vi "Read Section Cluster.vi"(6 "Section (Cluster Name)":string, 7 "error in (no error)":errorcluster, 8 "Cluster":variant, 9 "Offset":i32, 10 "JSON Object":string="{}") -> (0 "error out":errorcluster, 1 "Cluster set from section":variant, 2 "Section Found":bool)   [LabVIEW 2015, in "JSONtext.lvlib"]
doc: "Set the value of a Section Cluster from a Section of a JSON object. If the Section is not specified, then the data name of the Cluster will be used.\n\nA \"Section Cluster\" is defined in analogy to the OpenG Variant Config Library \"Section Cluster\" functions, using a JSON Object, with subObjects representing \"Sections\", instead of INI format."
uses:
  JSONtext.lvlib
  Find Object Item (single) by Path.vi
  String Subset.vi
  Find Item Locations by Path.vi
  JSON text to Variant.vi
  <vilib>/Utility/Data Type/NI_Data Type.lvlib
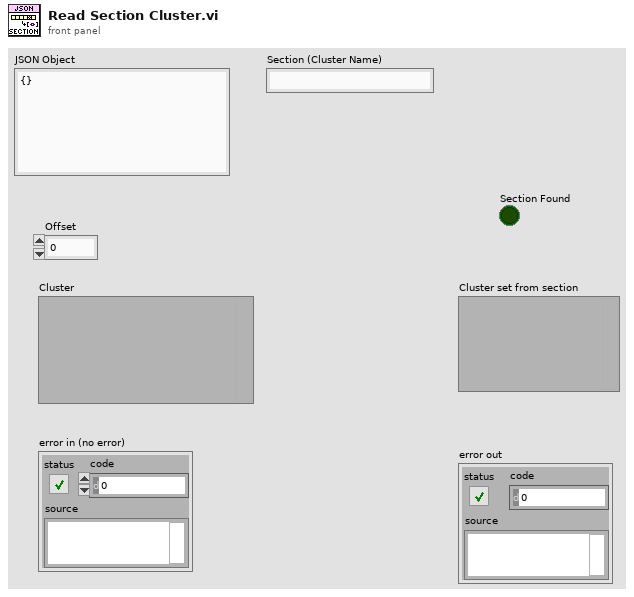
[diagram p1: front panel]
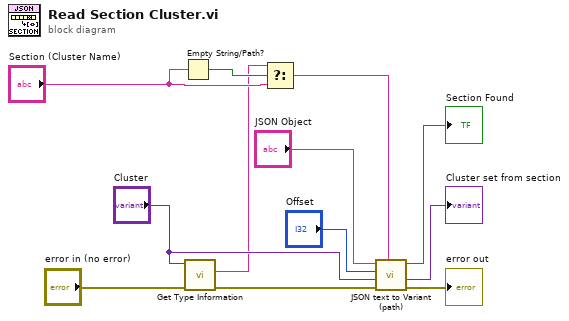
[diagram p0: block diagram]
diagram:
  n1 = Empty String/Path?(string/path="Section (Cluster Name)") -> (empty?=w4:bool)
  n2 = call <vilib>:"Get Type Information.vi"("error in (no error)"="error in (no error)", "Variant"="Cluster") -> ("error out"=w8:errorcluster, "Name"=w1:string)  [unwired: 5 in, 3 out]
  n3 = Select(t=w1, s=w4, f="Section (Cluster Name)") -> (s? t:f=w3:string)
  n4 = call "JSON text to Variant (path).vi"("Item Path"=w3, "error in (no error)"=w8, "Variant (Data Type)"="Cluster", "Starting Offset"="Offset", "JSON"="JSON Object") -> ("error out"=→"error out":errorcluster, "Variant out"=→"Cluster set from section":variant, "Found"=→"Section Found":bool)  [unwired: 4 in]
